vi "jog motor.vi"(8 "error in (no error)":errorcluster, 10 "CCW? (T)":bool=TRUE, 11 "CL57RS in":refnum<class "CL57RS.lvclass">) -> (0 "error out":errorcluster, 3 "CL57RS out":refnum<class "CL57RS.lvclass">)   [LabVIEW 2025, in "Motor.lvlib" / "CL57RS.lvclass"]
uses:
  CL57RS.lvclass
  CL57RS.lvclass/CL57RS.ctl
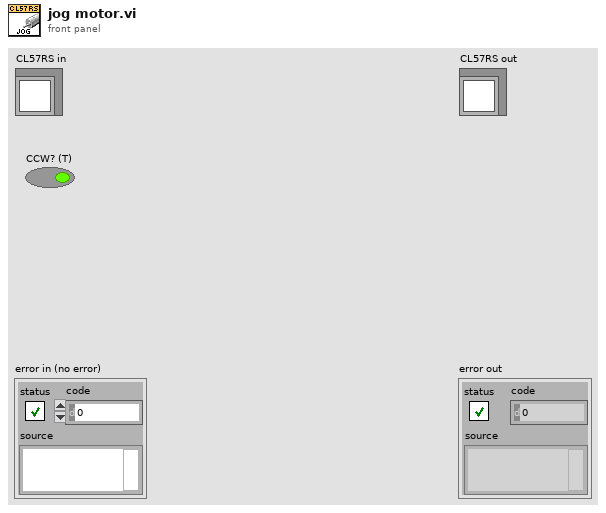
[diagram p1: front panel]
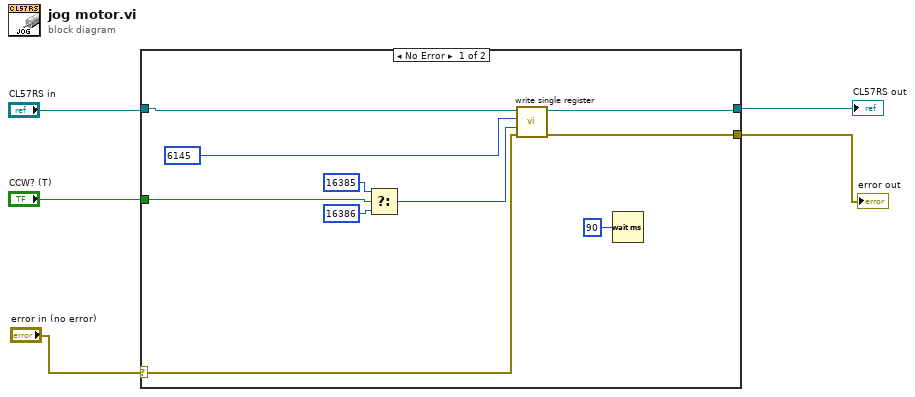
[diagram p0: block diagram]
diagram:
  n1 = case shown="No Error" "error in (no error)" {
    selector: "error in (no error)" -> [w12 w17]
    tunnel: [w13 w17] -> w1
    tunnel: [w14 w16] -> w4
    tunnel: "CL57RS in" -> [w15 w16]
    tunnel: "CCW? (T)" -> [w8 _]
    frame No Error {
      n2 = Select(t=u16 16385 ("address"), s=w8, f=u16 16386 ("address")) -> (s? t:f=w9:u16)
      n3 = call "write single register.vi"("error in (no error)"=w12, "register to write"=w9, "address"=u16 6145, "CL57RS in"=w15) -> ("error out"=w13:errorcluster, "CL57RS out"=w14:refnum<class "CL57RS.lvclass">)  [unwired: 6 in]
      n4 = Wait (ms)(milliseconds to wait=u32 90) -> ()  [unwired: 1 out]
    }
    frame Error {
    }
  }
  "error out" <- w1
  "CL57RS out" <- w4
